vi "CmdCode2Elements.vi"(1 "CommandCode":string) -> (0 "Elements":T1)   [LabVIEW 2010]
uses:
  <vilib>/regexp/Match Regular Expression.xnode
panel:
  out "whole match":string
  in  "regular expression":string="68[0-9ABCDEF]{12}68[0-9ABCDEF]{8,}16"
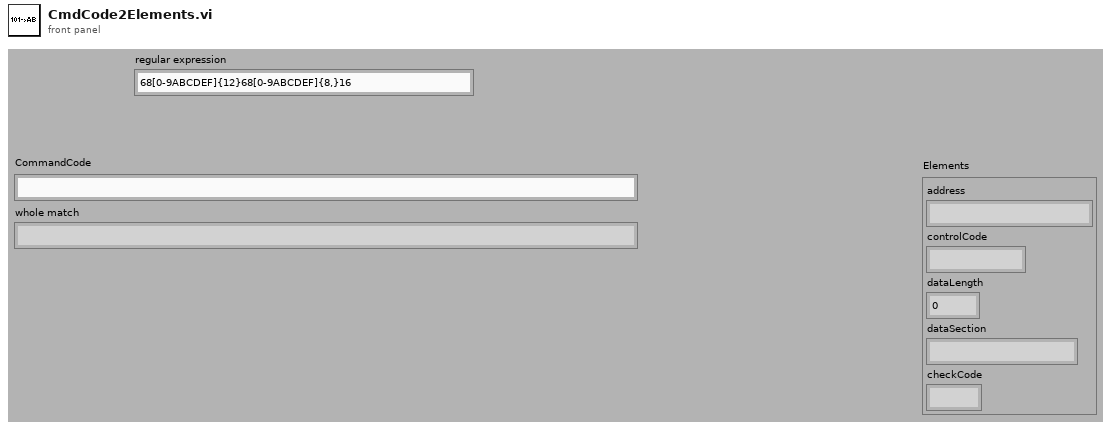
[diagram p1: front panel]
types:
  T1 = cluster{"address":string, "controlCode":string, "dataLength":dbl, "dataSection":string, "checkCode":string}
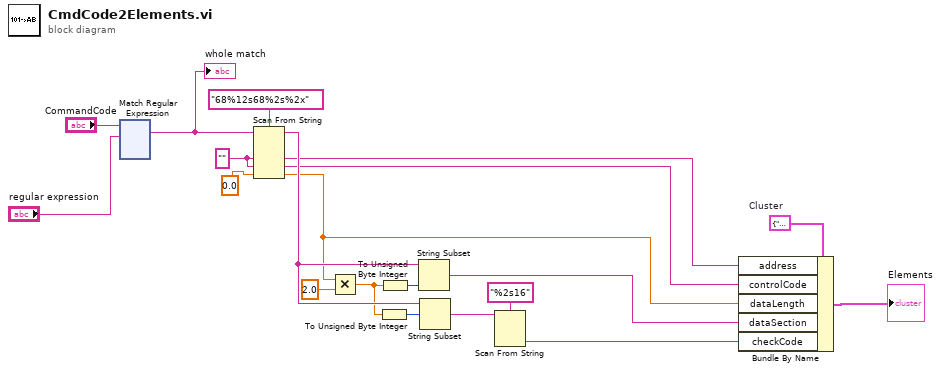
[diagram p0: block diagram]
diagram:
  w5 = T1 {"address"="100000000000", "controlCode"="15", "dataLength"=12.0, "dataSection"="343333333333", "checkCode"="47"}  # Cluster
  w17 = "" ("default value 1")
  n1 = xnode "Match Regular Expression"("input string"="CommandCode", "regular expression"="regular expression") -> ("whole match"=w18:string)  [unwired: 4 in, 4 out]
  "whole match" <- w18
  n2 = Scan From String(format string="68%12s68%2s%2x", input string=w18, default 1=w17, default 2=w17, default 3=0.0) -> (remaining string=w14:string, output 1=w9:string, output 2=w8:string, output 3=w7:dbl)  [unwired: 2 in, 2 out]
  n3 = Multiply(x=w7, y=2.0) -> (x*y=w2:dbl)
  n4 = To Unsigned Byte Integer(number=w2) -> (unsigned 8bit integer=w12:u8)
  n5 = To Unsigned Byte Integer(number=w2) -> (unsigned 8bit integer=w13:u8)
  n6 = String Subset(string=w14, length (rest)=w13) -> (substring=w3:string)  [unwired: 1 in]
  n7 = String Subset(string=w14, offset (0)=w12) -> (substring=w11:string)  [unwired: 1 in]
  n8 = Scan From String(format string="%2s16", input string=w11) -> (output 1=w6:string)  [unwired: 3 in, 3 out]
  n9 = Bundle By Name(cluster=w5, "address"=w9, "controlCode"=w8, "dataLength"=w7, "dataSection"=w3, "checkCode"=w6) -> (→"Elements":T1)
